vi "Set Needle Valve.vi"(8 "error in (no error)":errorcluster, 10 "Needle Valve (%)":dbl min=0.0 max=100.0, 11 "Instrument.1820 in":refnum<class "Instrument.OxfordVRM.lvclass">) -> (0 "error out":errorcluster, 2 "Response":string, 3 "Instrument.1820 in":refnum<class "Instrument.OxfordVRM.lvclass">)   [LabVIEW 2016, in "Instrument.OxfordVRM.lvclass"]
uses:
  Instrument.OxfordVRM.lvclass
  Typedefs/Instrument.Oxford1820.Commands-enum.ctl
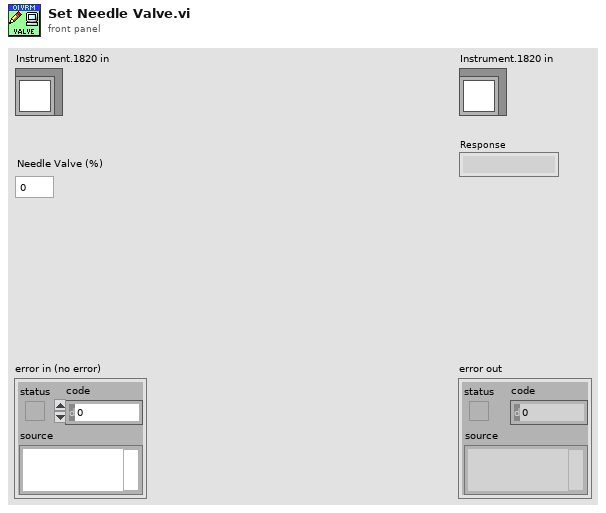
[diagram p1: front panel]
types:
  T1 = typedef "Instrument.OxfordVRM.lvclass/Instrument.Oxford1820.Commands-enum.ctl" = enum16{"setAction", "setTarget", "setSwitchHeat", "setLambda", "setFillMode", "setNeedleValve", "setMagnetField", "getStatus", "getTarget", "getSwitchHeat", "getPSUField", "newcommand", "getMagnetField"}
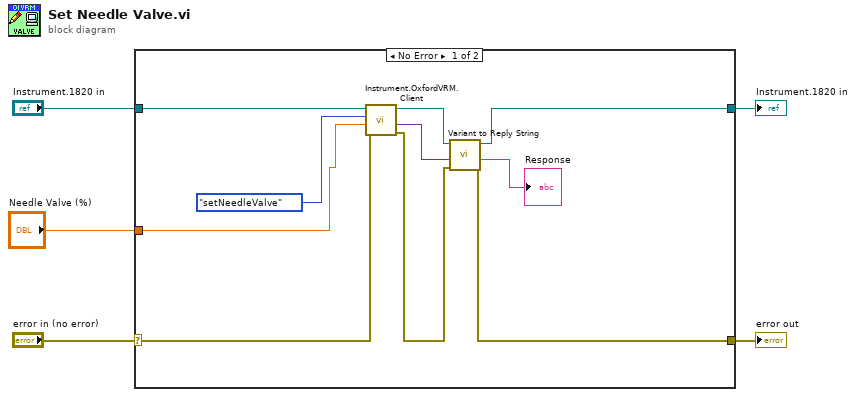
[diagram p0: block diagram]
diagram:
  n1 = case shown="No Error" "error in (no error)" {
    selector: "error in (no error)" -> [w14 w17]
    tunnel: [w8 w17] -> w4
    tunnel: [w6 w16] -> w2
    tunnel: "Instrument.1820 in" -> [w15 w16]
    tunnel: "Needle Valve (%)" -> [w12 _]
    frame No Error {
      n2 = call "Instrument.OxfordVRM.Client.vi"("error in (no error)"=w14, "Data"=w12, "Commands"=Instrument.Oxford1820.Commands-enum."setNeedleValve", "Instrument.1820 in"=w15) -> ("error out"=w9:errorcluster, "Data out"=w10:variant, "Instrument.1820 out"=w7:refnum<class "Instrument.OxfordVRM.lvclass">)  [unwired: 5 in]
      n3 = call "Variant to Reply String.vi"("error in (no error)"=w9, "Data"=w10, "Instrument.1820 in"=w7) -> ("error out"=w8:errorcluster, "Reply"=→"Response":string, "Instrument.1820 out"=w6:refnum<class "Instrument.OxfordVRM.lvclass">)  [unwired: 6 in]
    }
    frame Error {
    }
  }
  "error out" <- w4
  "Instrument.1820 in" <- w2
